vi "TagDB Refmgr-Remove.vi"(8 "error in (no error)":errorcluster, 10 "RegExp":string, 11 "TagDB in":refnum<k1>) -> (0 "error out":errorcluster, 1 "Keys":string[](array[string]), 2 "References":refnum<vi>[](array[refnum]), 3 "TagDB out":refnum<k1>)   [LabVIEW 2017, in "TagDB RefManager.lvlib"]
uses:
  TagDB RefManager.lvlib
  9d601a23-f96e-4540-83e7-41ff60b3d226.vi
  <userlib>/_NEVSTOP/TagDB/_Support/Change Detector/TagDB dbChanged.vi
  <userlib>/_NEVSTOP/TagDB/_Support/Error/_Clear Errors.vi
  9d601a23-f96e-4540-83e7-41ff60b3d226.vi/29b2ea6d-6d7f-4e4a-ad31-a5cb760462c7.vi
  <userlib>/_NEVSTOP/TagDB/API/TagDB-Status.vi
  <userlib>/_NEVSTOP/TagDB/_Support/Change Detector/TagDB ChangeFlag.vi
  <userlib>/_NEVSTOP/TagDB/_Support/DataAccess/_NameCacher.vi
  <userlib>/_NEVSTOP/TagDB/_Support/Error/_[error50002]Invalid DataType.vi
  <userlib>/_NEVSTOP/TagDB/_Support/Error/_[error50000]Invalid DB REF.vi
  <userlib>/_NEVSTOP/TagDB/_Support/DataAccess/TagDB Ref to DVR.vi
  <userlib>/_NEVSTOP/TagDB/_Support/URL/TRIM-BOTH-SPACE.vi
  <userlib>/_NEVSTOP/TagDB/API/TagDB-Delete Multiple.vi
  <userlib>/_NEVSTOP/TagDB/_Support/Error/_Build Error Cluster.vi
  <userlib>/_NEVSTOP/TagDB/TagDB.lvlib
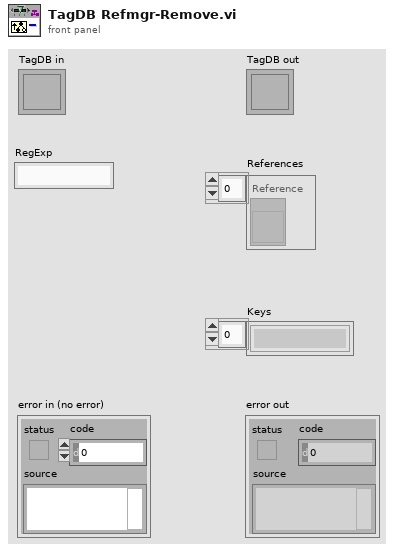
[diagram p1: front panel]
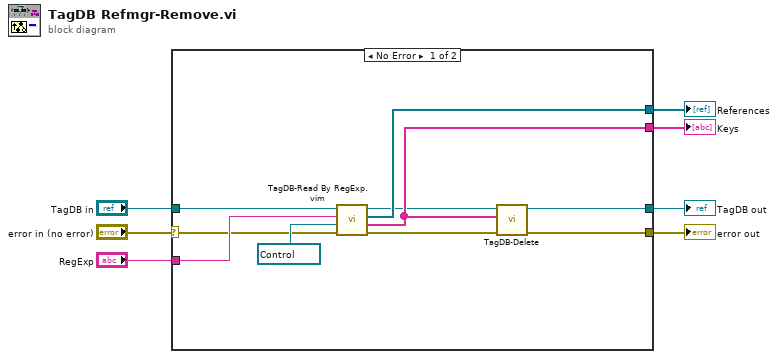
[diagram p0: block diagram]
diagram:
  n1 = case shown="No Error" "error in (no error)" {
    selector: "error in (no error)" -> [w8 w19]
    tunnel: "RegExp" -> [w17 _]
    tunnel: [w16 _] -> w6
    tunnel: [w15 _] -> w5
    tunnel: "TagDB in" -> [w11 w18]
    tunnel: [w10 w18] -> w3
    tunnel: [w9 w19] -> w2
    frame No Error {
      n2 = call "TagDB-Read By RegExp.vim"("error in (no error)"=w8, "Type"=refnum<vi> refnum, "RegExp"=w17, "DB Ref"=w11) -> ("error out"=w12:errorcluster, "names"=w15:string[], "value"=w16:refnum<vi>[], "DB Ref(dup)"=w13:refnum<k1>)  [unwired: 4 in]
      n3 = call-poly <userlib>:"TagDB-Delete.vi"("error in (no error)"=w12, "Tags"=w15, "TagDB"=w13) -> ("error out"=w9:errorcluster, "TagDB(dup)"=w10:refnum<k1>)  [unwired: 7 in]
    }
    frame Error {
    }
  }
  "References" <- w6
  "Keys" <- w5
  "error out" <- w2
  "TagDB out" <- w3
